vi "Irregular_Wave_Generation.vi"() -> ()   [LabVIEW 2018]
panel:
  in  "Knob":dbl(knob) scale=0.0..2.0
  out "Waveform Chart 2":dynamicdata(graph)
  in  "Wave Type Selector":bool
  out "Time Series Length":dbl
  in  "Number Waves  \nto generate":dbl=100.0
  in  "Wave Period [s]":dbl=1.0
  in  "Wave Height [cm]":dbl=5.0
  out "Run Errors":errorcluster
  out "Output Voltage":dbl(graph)
  in  "Start Wave Generation":bool
  in  "stop":bool
  in  "Bias Voltage":dbl=3.0 min=-0.2 max=0.0 step=0.01
  out "Mean Paddle Stroke":dbl
  out "Min Paddle Displacement":dbl
  out "Max Paddle Displacement":dbl
  in  "Number of Peak Waves":dbl=100.0
  in  "Peak Spectral Period\n[s]":dbl=1.0
  in  "Significant Wave Height\n[cm]":dbl=5.0
  in  "Water Depth\n[m]":dbl=1.5
  # "Irregular Sea State Constraints"
  # "Periodic Wave Constraints"
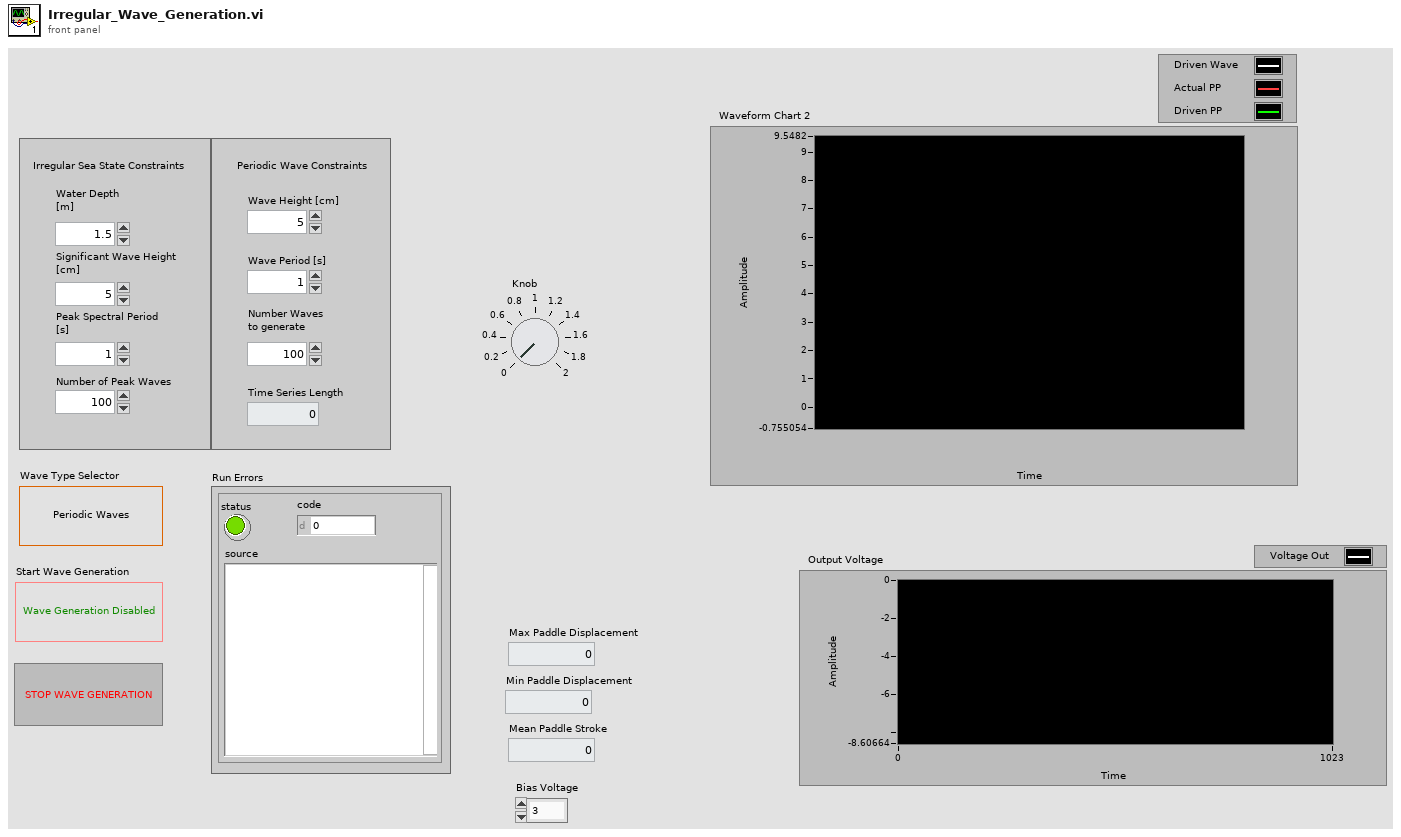
[diagram p1: front panel]
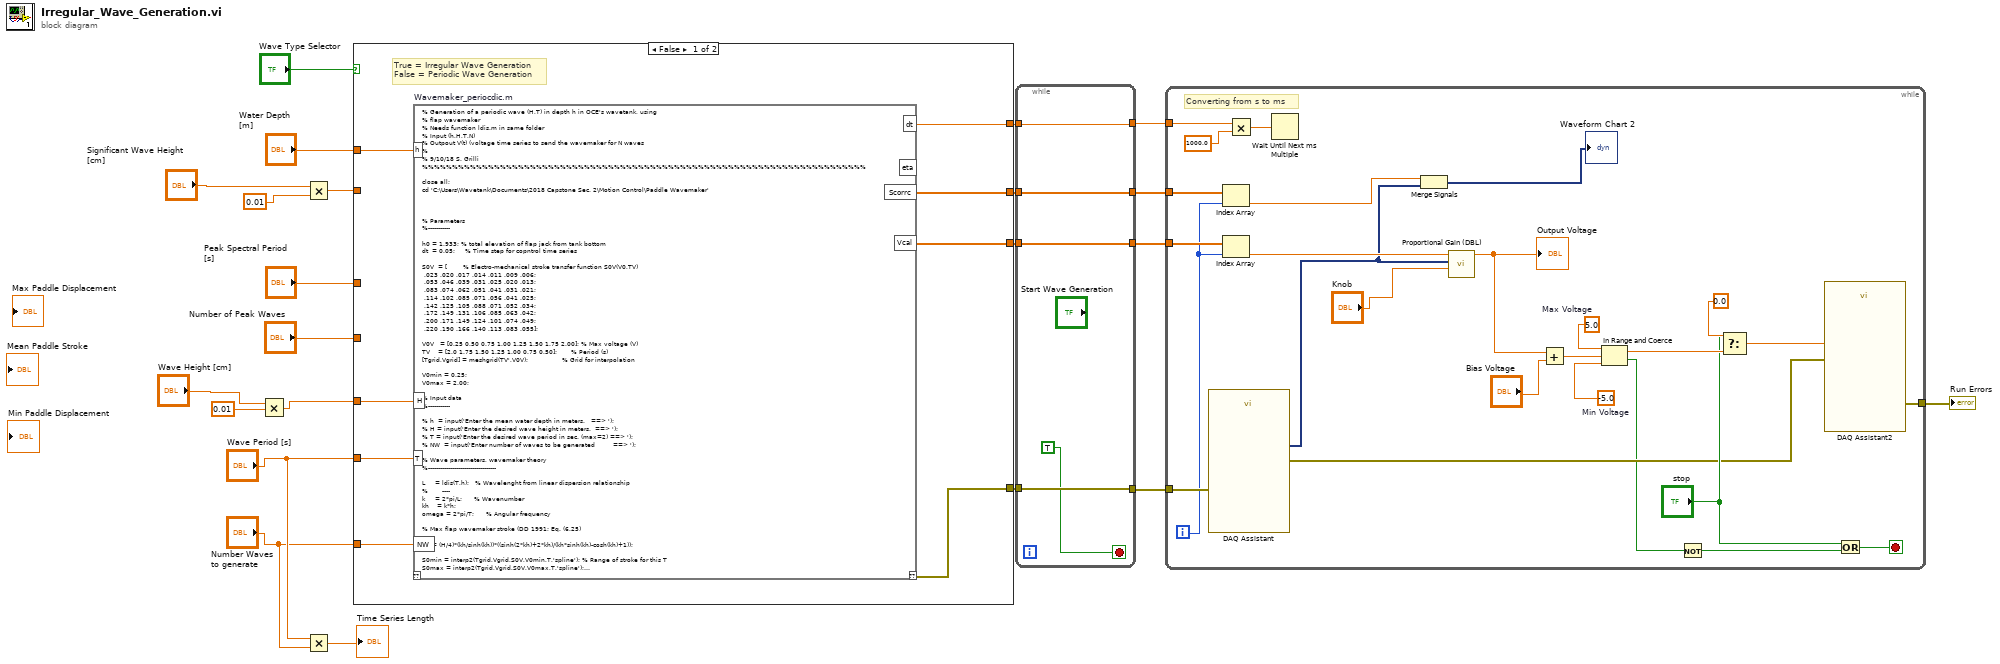
[diagram p0: block diagram]
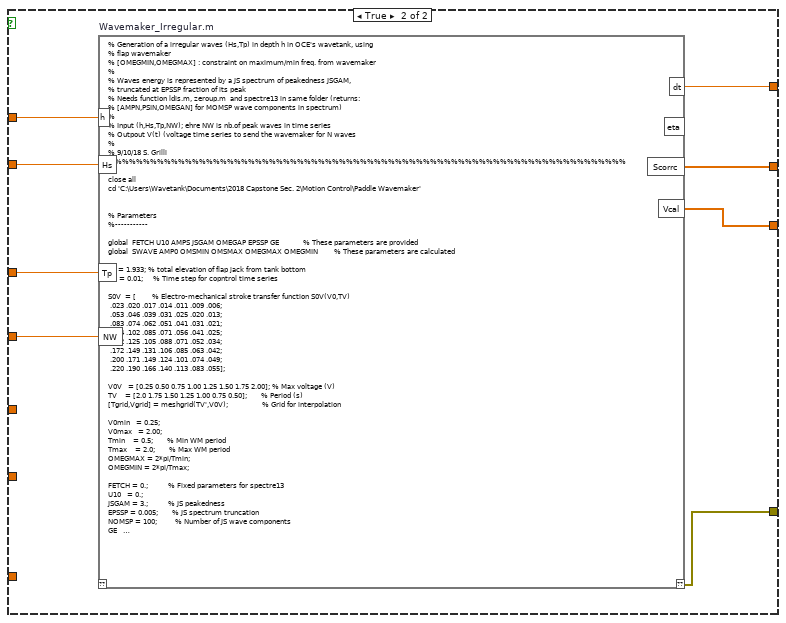
[diagram p2: hidden frame]
diagram:
  n1 = Multiply(x="Wave Height [cm]", y=0.01) -> (x*y=w1:dbl)
  n2 = Multiply(x="Significant Wave Height\n[cm]", y=0.01) -> (x*y=w4:dbl)
  n3 = Multiply(x="Wave Period [s]", y="Number Waves  \nto generate") -> (x*y=→"Time Series Length":dbl)
  n4 = case shown="False" "Wave Type Selector" {
    tunnel: "Number of Peak Waves" -> [_ w38]
    tunnel: "Peak Spectral Period\n[s]" -> [_ w37]
    tunnel: "Water Depth\n[m]" -> [w30 w36]
    tunnel: w4 -> [_ w35]
    tunnel: [w29 w34] -> w19
    tunnel: [w28 w33] -> w16
    tunnel: [w27 w32] -> w15
    tunnel: [w23 w31] -> w14
    tunnel: "Number Waves  \nto generate" -> [w26 _]
    tunnel: "Wave Period [s]" -> [w25 _]
    tunnel: w1 -> [w24 _]
    frame False {
      # "True = Irregular Wave Generation\nFalse = Periodic Wave Generation"
      n5 = script code="% Generation of a periodic wave (H,T) in depth h in OCE's wavetank, using\n% flap wavemaker\n% Needs function ldis.m in same folder\n% Input (h,H,T,N)\n% Outpout V(t) (voltage time series to send the wavemaker for N waves\n%\n% 9/10/18 S. Grilli\n%%%%%%%%%%%%%%%%%%%%%%%%%%%%%%%%%%%%%%%%%%%%%%%%%%%%%%%%%%%%%%%%%%%%%%%%%%\n\nclose all; \ncd 'C:\\Users\\Wavetank\\Documents\\2018 Capstone Sec. 2\\Motion Control\\Paddle Wavemaker'\n\n\n\n% Parameters\n%-----------\n\nh0\t= 1.933;\t% total elevation of flap jack from tank bottom\ndt  = 0.05;     % Time step for copntrol time series\n\nS0V  = [        % Electro-mechanical stroke transfer function S0V(V0,TV)\n .023 .020 .017 .014 .011 .009 .006;\n .053 .046 .039 .031 .025 .020 .013;\n .083 .074 .062 .051 .041 .031 .021;\n .114 .102 .085 .071 .056 .041 .025;\n .142 .125 .105 .088 .071 .052 .034;\n .172 .149 .131 .106 .085 .063 .042;\n .200 .171 .149 .124 .101 .074 .049;\n .220 .190 .166 .140 .113 .083 .055];\n\nV0V   = [0.25 0.50 0.75 1.00 1.25 1.50 1.75 2.00]; % Max voltage (V) \nTV    = [2.0 1.75 1.50 1.25 1.00 0.75 0.50];       % Period (s)\n[Tgrid,Vgrid] = meshgrid(TV',V0V);                 % Grid for interpolation\n\nV0min = 0.25;\nV0max = 2.00;\n\n% Input data\n%-----------\n\n% h \t= input('Enter the mean water depth in meters.\t\t\t==> ');\n% H\t= input('Enter the desired wave height in meters.\t\t==> ');\n% T\t= input('Enter the desired wave period in sec. (max=2)\t==> ');\n% NW  = input('Enter number of waves to be generated\t        ==> ');\n\n% Wave parameters, wavemaker theory\n%----------------------------------\n\nL     = ldis(T,h);   % Wavelenght from linear dispersion relationship\n%       ----\nk     = 2*pi/L;      % Wavenumber\nkh    = k*h;\nomega = 2*pi/T;      % Angular frequency\n\n% Max flap wavemaker stroke (DD 1991; Eq. (6.25)\n\nS0 = (H/4)*(kh/sinh(kh))*((sinh(2*kh)+2*kh)/(kh*sinh(kh)-cosh(kh)+1));\n\nS0min = interp2(Tgrid,Vgrid,S0V,V0min,T,'spline'); % Range of stroke for this T\nS0max = interp2(Tgrid,Vgrid,S0V,V0max,T,'spline');\n\nif (S0 > S0max) \n    H = input('Stroke too large for this T. Enter a smaller wave height ==> ');\nend\nif (S0 < S0min) \n    H = input('Stroke too small for this T. Enter a larger wave height ==> ');\nend\n\n% Max voltage interpolated for WM\n%--------------------------------\n\nS0T(:) = interp2(Tgrid,Vgrid,S0V,V0V(:),T,'spline'); % Range of stroke for this T\nq      = polyfit(S0T,V0V,3);  %  Curve fit V(S) for given T values\nV0     = polyval(q,S0)  %  Max voltage for Wavemaker control law\n\n% Voltage timne series sent to wavemaker\n%--------------------------------------\n\ntmax = T*NW;\nt    = 0:dt:tmax;\nNt   = length(t);\nV    = 0.5*V0*(1 - cos(omega*t));\n\nfigure(1)\nplot(t,V,'-b','LineWidth',1.5)\ngrid on\nxlabel('t (s)','Fontsize',20);\nylabel('V (V)','Fontsize',20);\ntitle(['Voltage time series (H = ' num2str(H) ' m ; h = ' num2str(h) ' m ; T = ' num2str(T) ' s)'],'Fontsize',20);\nset(gca,'FontSize',20);" "Wavemaker_periocdic.m"("h"=w30, "H"=w24, "NW"=w26, "T"=w25) -> ("??"=w23:errorcluster, "Scorrc"=w28:dbl[], "Vcal"=w27:dbl[], "dt"=w29:dbl)  [unwired: 1 in, 1 out]
    }
    frame True {
      n6 = script code="% Generation of a irregular waves (Hs,Tp) in depth h in OCE's wavetank, using\n% flap wavemaker\n% [OMEGMIN,OMEGMAX] : constraint on maximum/min freq. from wavemaker\n%\n% Waves energy is represented by a JS spectrum of peakedness JSGAM,\n% truncated at EPSSP fraction of its peak\n% Needs function ldis.m, zeroup.m  and spectre13 in same folder (returns:\n% [AMPN,PSIN,OMEGAN] for MOMSP wave components in spectrum)\n%\n% Input (h,Hs,Tp,NW); ehre NW is nb.of peak waves in time series\n% Outpout V(t) (voltage time series to send the wavemaker for N waves\n%\n% 9/10/18 S. Grilli\n%%%%%%%%%%%%%%%%%%%%%%%%%%%%%%%%%%%%%%%%%%%%%%%%%%%%%%%%%%%%%%%%%%%%%%%%%%\n\nclose all\ncd 'C:\\Users\\Wavetank\\Documents\\2018 Capstone Sec. 2\\Motion Control\\Paddle Wavemaker'\n\n\n% Parameters\n%-----------\n\nglobal  FETCH U10 AMPS JSGAM OMEGAP EPSSP GE            % These parameters are provided\nglobal  SWAVE AMP0 OMSMIN OMSMAX OMEGMAX OMEGMIN        % These parameters are calculated\n\nh0\t= 1.933;\t% total elevation of flap jack from tank bottom\ndt  = 0.01;     % Time step for copntrol time series\n\nS0V  = [        % Electro-mechanical stroke transfer function S0V(V0,TV)\n .023 .020 .017 .014 .011 .009 .006;\n .053 .046 .039 .031 .025 .020 .013;\n .083 .074 .062 .051 .041 .031 .021;\n .114 .102 .085 .071 .056 .041 .025;\n .142 .125 .105 .088 .071 .052 .034;\n .172 .149 .131 .106 .085 .063 .042;\n .200 .171 .149 .124 .101 .074 .049;\n .220 .190 .166 .140 .113 .083 .055];\n\nV0V   = [0.25 0.50 0.75 1.00 1.25 1.50 1.75 2.00]; % Max voltage (V) \nTV    = [2.0 1.75 1.50 1.25 1.00 0.75 0.50];       % Period (s)\n[Tgrid,Vgrid] = meshgrid(TV',V0V);                 % Grid for interpolation\n\nV0min   = 0.25;\nV0max   = 2.00;\nTmin    = 0.5;       % Min WM period\nTmax    = 2.0;       % Max WM period\nOMEGMAX = 2*pi/Tmin;\nOMEGMIN = 2*pi/Tmax;\n\nFETCH = 0.;          % Fixed parameters for spectre13\nU10   = 0.;\nJSGAM = 3.;          % JS peakedness\nEPSSP = 0.005;       % JS spectrum truncation\nNOMSP = 100;         % Number of JS wave components\nGE    = 9.81;\n\n% Input data\n%-----------\n\n%h \t= input('Enter the mean water depth in meters.\t     ==> ');\n%Hs\t= input('Enter the significant wave height (m)       ==> ');\n%Tp\t= input('Enter the peak spectral period (s) (max=2)\t ==> ');\n%NW  = input('Enter number of peak waves to be generated\t ==> ');\n\nAMPS   = Hs/2;\nOMEGAP = 2*pi/Tp;\n\n% Generates JS spectrum and wave harmonics\n%-----------------------------------------\n\n[AMPN,PSIN,OMEGAN] = spectre13(NOMSP);\n%                    ---------\nHs0 = 2*AMP0;\nfmin = OMSMIN/(2*pi);\nfmax = OMSMAX/(2*pi);\nTN   = 2*pi./OMEGAN;\n\nfigure(1)\nplot(OMEGAN/(2*pi),SWAVE); % spectral amplitude plot\ntitle(['Ocean wave spectrum' ' H_{s0}=' num2str(Hs0) ' m, T_p=' num2str(Tp) ' s'],...\n           'fontsize',16);    \nxlabel('f (Hz)','fontsize',16);\nylabel('S (m^2. s)','fontsize',16);\ngrid on;\nNOM = NOMSP;\n\n% Wave parameters, wavemaker theory\n%----------------------------------\n\nLN    = ldis(TN,h);  % Wavelenght from linear dispersion relationship\n%       ----\nkN    = 2*pi./LN;      % Wavenumber\nkNh   = kN*h;\n\n% Max flap wavemaker stroke corrected for elevation (DD 1991; Eq. (6.25))\n\nS0N = (h0/h)*(AMPN/2).*(kNh./sinh(kNh)).*((sinh(2*kNh)+ 2*kNh)./(kNh.*sinh(kNh)-cosh(kNh)+1));\n\n% Stroke time series for WM \n%---------------------------\n\ntmax = Tp*NW;\nt    = 0:dt:tmax;\nNt   = length(t);\n\n% Wave time series targeted in tank\n\nfor it = 1:Nt\n    eta(it) = 0.5*sum(AMPN(:).*(cos(OMEGAN(:)*t(it) + PSIN(:))));\nend\n\nfigure(2)\nplot(t,eta,'-b','LineWidth',1.5)\ngrid on\nxlabel('t (s)','Fontsize',20);\nylabel('\\eta (m)','Fontsize',20);\ntitle(['Wave time series (H_s = ' num2str(Hs) ' m ; h = ' num2str(h) ' m ; T_p = ' num2str(Tp) ' s)'],'Fontsize',20);\nset(gca,'FontSize',20);\n\n% Theoretical stroke time series\n\nfor it = 1:Nt\n    S(it) = 0.5*sum(S0N(:).*(1 - cos(OMEGAN(:)*t(it) + PSIN(:))));\nend\n\nSmean = mean(S);  % Demean stroke for ZUC\nScorr = S - Smean;\n\nfigure(3)\nplot(t,Scorr,'-b','LineWidth',1.5)\ngrid on\nxlabel('t (s)','Fontsize',20);\nylabel('S (m)','Fontsize',20);\ntitle(['Stroke time series (H_s = ' num2str(Hs) ' m ; h = ' num2str(h) ' m ; T_p = ' num2str(Tp) ' s)'],'Fontsize',20);\nset(gca,'FontSize',20);\n\n% ZUC analysis opf stroke time series\n%------------------------------------\n\njzuc    = 0;\nNst     = 0;\nScmax   = 0;\nScmin   = 0;\ntstart  = 0;\n\nfor it = 1:Nt-1\n    Scmax = max(Scorr(it),Scmax);\n    Scmin = min(Scorr(it),Scmin);\n    \n    if (Scorr(it) < 0) & (Scorr(it+1) >= 0)  % ZUC\n        jzuc       = jzuc + 1; \n        izuc(jzuc) = it;\n        tend(jzuc) = t(it) + (dt/(Scorr(it+1)-Scorr(it)))*Scorr(it+1);\n        Sper(jzuc) = tend(jzuc) - tstart;\n        tstart     = tend(jzuc);\n        Sint(jzuc) = Scmax - Scmin;\n        Nst         = Nst + 1;\n        Scmax      = 0;\n        Scmin      = 0;\n    end\nend\n\n% Enforces lower and upper bound on stroke based on wavemaker stroke function\n\nfor n=2:Nst\n    Sfin(n-1) = Sint(n);  % Shift to the first ZUC\n    \n    S0min  = interp1(TV,S0V(1,:),Sper(n),'spline'); % Min stroke for this T, Vmin\n    S0max  = interp1(TV,S0V(8,:),Sper(n),'spline'); % Max stroke for this T, Vmax\n\n    if (Sint(n) > S0max) \n        Sfin(n-1) = S0max;\n    end\n    if (Sint(n) < S0min) \n        Sfin(n-1) = S0min;\n    end\nend\n\nSTfin  = Sper(2:Nst);\ntstr   = t(izuc) - t(izuc(1));              % beginning and end of each stroke\ntcor   = t(izuc(1):izuc(Nst))- t(izuc(1));  % new time series\nScorr0 = Scorr(izuc(1):izuc(Nst));          % new stroke time series\nNst    = Nst-1;                             % Nb. of strokes\nNtc    = length(tcor);\n\nfigure(31)\nplot(tcor,Scorr0,'-b','LineWidth',1.5)\ngrid on\nxlabel('t (s)','Fontsize',20);\nylabel('S (m)','Fontsize',20);\ntitle(['Stroke time series (H_s = ' num2str(Hs) ' m ; h = ' num2str(h) ' m ; T_p = ' num2str(Tp) ' s)'],'Fontsize',20);\nset(gca,'FontSize',20);\n\n% Max voltage for each (trough to crest) stroke in ZUC analysis\n\nfor n=1:Nst\n    S0T(:) = interp2(Tgrid,Vgrid,S0V,V0V(:),STfin(n),'spline'); % Range of stroke for this JS spectrum\n    q      = polyfit(S0T,V0V,3);   %  Curve fit V(S) for given T values\n    V0(n)  = polyval(q,Sfin(n));   %  Max voltage for Wavemaker control law\nend\n\nV0all = [0 V0];\nV0fit = interp1(tstr,V0all,tcor);   %  Curve fit V0(strokes) \n\nfigure(4)\nplot(tstr,V0all,'-b',tcor,V0fit,'-r','LineWidth',1.5)\ngrid on\nxlabel('t (s)','Fontsize',20);\nylabel('V (V)','Fontsize',20);\ntitle(['Max voltage time series (H_s = ' num2str(Hs) ' m ; h = ' num2str(h) ' m ; T_p = ' num2str(Tp) ' s)'],'Fontsize',20);\nset(gca,'FontSize',20);\n\n% Voltage timne series with random phase, to be sent to wavemaker\n%----------------------------------------------------------------\n\nSfac = Sint(2);\niac  = 1;\nit   = 1;\n\nwhile (it <= Ntc) & (iac <= Nst)    \n    if tcor(it) > tstr(iac+1)\n        iac = iac + 1;\n        Sfac = Sint(iac+1);\n    end\n    Scorrc(it) = Scorr0(it)/Sfac;\n    Vcal(it)   = V0fit(it)*Scorrc(it);\n    it = it + 1;\nend\n\n%figure(5)\n%plot(tcor,Vcal,'-b','LineWidth',1.5)\n%grid on\n%xlabel('t (s)','Fontsize',20);\n%ylabel('V (V)','Fontsize',20);\n%title(['Voltage time series (H_s = ' num2str(Hs) ' m ; h = ' num2str(h) ' m ; T_p = ' num2str(Tp) ' s)'],'Fontsize',20);\n%set(gca,'FontSize',20);\n\n%figure(6)\n%plot(tcor,Scorrc,'-b','LineWidth',1.5)\n%grid on\n%xlabel('t (s)','Fontsize',20);\n%ylabel('Sc (m)','Fontsize',20);\n%title(['Stroke time series (H_s = ' num2str(Hs) ' m ; h = ' num2str(h) ' m ; T_p = ' num2str(Tp) ' s)'],'Fontsize',20);\n%set(gca,'FontSize',20);" "Wavemaker_Irregular.m"("h"=w36, "Hs"=w35, "NW"=w38, "Tp"=w37) -> ("??"=w31:errorcluster, "Scorrc"=w33:dbl[], "Vcal"=w32:dbl[], "dt"=w34:dbl)  [unwired: 1 in, 1 out]
    }
  }
  n7 = while {
    tunnel: [w43] -> w18
    tunnel: w19 -> [w43]
    tunnel: [w42] -> w17
    tunnel: w16 -> [w42]
    tunnel: [w41] -> w13
    tunnel: w15 -> [w41]
    tunnel: [w40] -> w12
    tunnel: w14 -> [w40]
    stop <- TRUE stop-if-true
  }
  n8 = while {
    tunnel: w12 -> [w69]
    tunnel: w18 -> [w57]
    tunnel: w17 -> [w68]
    tunnel: w13 -> [w61]
    tunnel: [w52] -> w11
    i -> [w60]
    stop <- w49 stop-if-true
    w65 = 5.0  # Max Voltage
    w66 = -5.0  # Min Voltage
    # "Converting from s to ms"
    n9 = call "DAQ Assistant"("error in"=w69) -> ("data"=w46:dynamicdata, "error out"=w53:errorcluster)  [unwired: 16 in, 1 out]
    n10 = Index Array(array=w68, index=w60) -> (element=w47:dbl)
    n11 = Index Array(array=w61, index=w60) -> (element=w59:dbl)
    n12 = Multiply(x=w57, y=1000.0) -> (x*y=w56:dbl)
    n13 = Wait Until Next ms Multiple(millisecond multiple=w56) -> ()  [unwired: 1 out]
    n14 = Merge Signals(w47, w46) -> (→"Waveform Chart 2":dynamicdata)
    n15 = call "Proportional Gain (DBL).vi"("Proportional Gain"="Knob", "Process Variable"=w46, "Set Point"=w59) -> ("Output Value"=w54:dbl)  [unwired: 8 in]
    "Output Voltage" <- w54
    n16 = Add(x=w54, y="Bias Voltage") -> (x+y=w64:dbl)
    n17 = In Range and Coerce(upper limit=w65, x=w64, lower limit=w66) -> (coerced(x)=w63:dbl, In Range?=w51:bool)
    n18 = Not(x=w51) -> (.not. x?=w50:bool)
    n19 = Select(t=0.0, s="stop", f=w63) -> (s? t:f=w48:dbl)
    n20 = call "DAQ Assistant2"("data"=w48, "error in"=w53) -> ("error out"=w52:errorcluster)  [unwired: 16 in, 1 out]
    n21 = Or(x="stop", y=w50) -> (x .or. y?=w49:bool)
  }
  "Run Errors" <- w11
